vi "ExSubAsyncColDispStore.vi"(2 "error in (no error)":errorcluster, 3 "Store Data":bool, 4 "Display Title":string, 5 "Handle Cluster":T1) -> (0 "error out":errorcluster, 1 "Handle Cluster Out":T1)   [LabVIEW 2010]
panel:
  # "ExSubAsyncColDispStore:\nThis Sub-VI collects imageas in Async mode\nwhich means a start before every frame. It \nthen checks to see if data has arrived, if so it\ndisplays it and if store toggle is on will store in\nin a file."
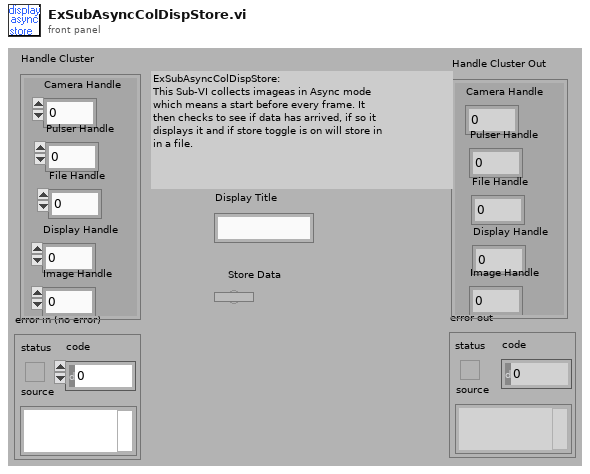
[diagram p1: front panel]
types:
  T1 = cluster{"Camera Handle":u32, "Pulser Handle":u32, "File Handle":u32, "Display Handle":u32, "Image Handle":u32}
  T2 = cluster{"Camera Handle":u32, "Pulser Handle":u32, "File Handle":u32, "Display Handle":u32, "Data Handle":u32}
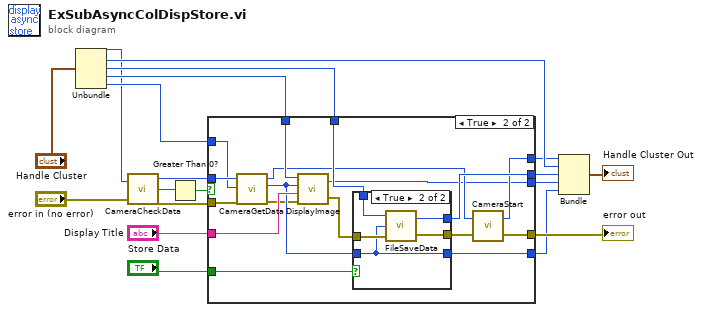
[diagram p0: block diagram]
diagram:
  n1 = Unbundle("Handle Cluster") -> ("Camera Handle"=w5:u32, "Pulser Handle"=w8:u32, "File Handle"=w9:u32, "Display Handle"=w11:u32, "Image Handle"=w12:u32)
  n2 = call <userlib>:"CameraCheckData.vi"("Camera Handle"=w5, "error in"="error in (no error)") -> ("Camera Handle"=w16:u32, "Number Of Frames Available"=w15:i32, "error out"=w14:errorcluster)
  n3 = Greater Than 0?(x=w15) -> (x > 0?=w17:bool)
  n4 = case shown="True" w17 {
    tunnel: w16 -> [w24 w41]
    tunnel: w14 -> [w23 w40]
    tunnel: w12 -> [w20 w38]
    tunnel: w11 -> [w22 w37]
    tunnel: [w24 w27] -> w6
    tunnel: [w21 w39] -> w4
    tunnel: "Display Title" -> [_ w36]
    tunnel: w9 -> [w21 w35]
    tunnel: [w22 w25] -> w3
    tunnel: [w23 w28] -> w7
    tunnel: [w20 w33] -> w2
    tunnel: "Store Data" -> [_ w32]
    frame False {
    }
    frame True {
      n5 = call <userlib>:"CameraGetData.vi"("error in"=w40, "Data Handle"=w38, "Camera Handle"=w41) -> ("error out"=w31:errorcluster, "Data Handle"=w34:u32, "Camera Handle"=w26:u32)
      n6 = call <userlib>:"DisplayImage.vi"("error in"=w31, "Title"=w36, "Image Handle"=w34, "Display Handle"=w37) -> ("error out"=w30:errorcluster, "Display Handle"=w25:u32)
      n7 = case shown="True" w32 {
        tunnel: [w44 w49] -> w39
        tunnel: w30 -> [w43 w48]
        tunnel: w35 -> [w44 w46]
        tunnel: [w43 w47] -> w29
        tunnel: w34 -> [w42 w45]
        tunnel: [w42 w45] -> w33
        frame False {
        }
        frame True {
          n8 = call <userlib>:"FileSaveData.vi"("error in"=w48, "Image Handle"=w45, "File Handle"=w46) -> ("error out"=w47:errorcluster, "File Handle"=w49:u32)
        }
      }
      n9 = call <userlib>:"CameraStart.vi"("error in"=w29, "Camera Handle"=w26) -> ("error out"=w28:errorcluster, "Camera Handle"=w27:u32)
    }
  }
  "error out" <- w7
  n10 = Bundle("Camera Handle"=w6, "Pulser Handle"=w8, "File Handle"=w4, "Display Handle"=w3, "Data Handle"=w2) -> (→"Handle Cluster Out":T2)  [unwired: 1 in]
